vi "16pxBlackOpenFile.vi"() -> (3 "OpenFileWhite":refnum<class "Image.lvclass">)   [LabVIEW 2021, in "Menu.lvlib" / "Menu.lvclass"]
uses:
  Menu.lvclass
  Menu.lvclass/Menu.ctl
  Picture2D/src/Picture/Image.lvclass
  Picture2D/src/Point/Point.lvclass
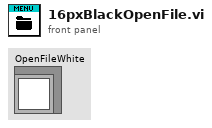
[diagram p1: front panel]
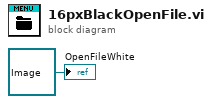
[diagram p0: block diagram]
diagram:
  "OpenFileWhite" <- refnum<class "Image.lvclass"> refnum ("Image out")
